vi "DSF.Engine.Memory.Cache.Transfer.Create.vi"(8 "error in (no error)":errorcluster, 10 "Transfer Configuration":refnum<class "DSF.Shared.Configuration.Transfer.lvclass">, 11 "Transfer Cache type":refnum<class "DSF.Engine.Memory.Cache.Transfer.lvclass">) -> (0 "error out":errorcluster, 3 "Transfer Cache":refnum<class "DSF.Engine.Memory.Cache.Transfer.lvclass">)   [LabVIEW 2016, in "DSF.Engine.lvlib" / "DSF.Engine.Memory.Cache.Transfer.lvclass"]
uses:
  DSF.Engine.Memory.Cache.Transfer.lvclass
  Shared/Classes/Transfer/DSF.Shared.Configuration.Transfer.lvclass
  DSF.Engine.Memory.Cache.Transfer.lvclass/DSF.Engine.Memory.Cache.Transfer.ctl
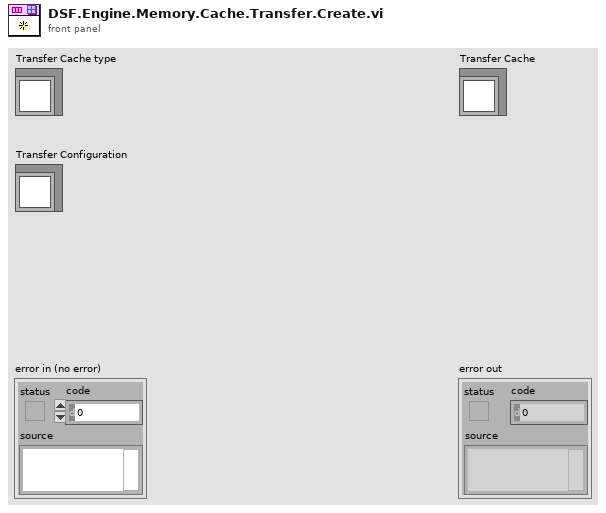
[diagram p1: front panel]
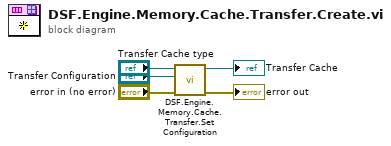
[diagram p0: block diagram]
diagram:
  n1 = call "DSF.Engine.Memory.Cache.Transfer.Set Configuration.vi"("Transfer Configuration"="Transfer Configuration", "Transfer Cache in"="Transfer Cache type") -> ("Transfer Cache out"=→"Transfer Cache":refnum<class "DSF.Engine.Memory.Cache.Transfer.lvclass">)  [unwired: 9 in]
  "error out" <- "error in (no error)"
